vi "RT testbead.vi"() -> ()   [LabVIEW 2009]
uses:
  <vilib>/Instr/_visa.llb/VISA Configure Serial Port (Instr).vi
  behaviors/driveable path/drivable paths global.vi
panel:
  out "driveable path lengths (lines)":u16[](array[numeric])
  out "Serial Settings:Number of Bytes at Serial Port":u32
  in  "stop":bool
  out "read buffer":string
  in  "VISA resource name":refnum<visa-resource-name>
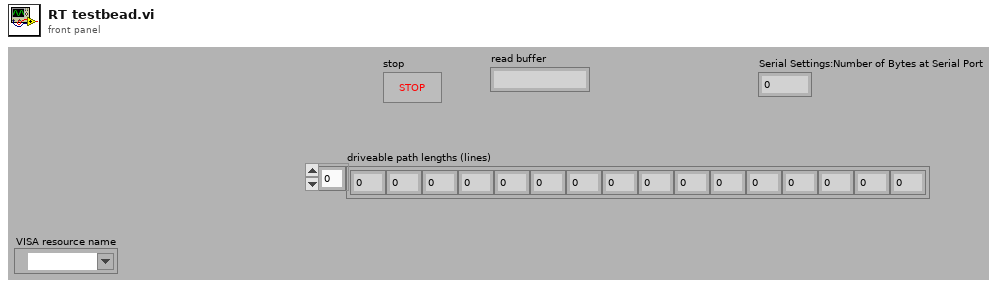
[diagram p1: front panel]
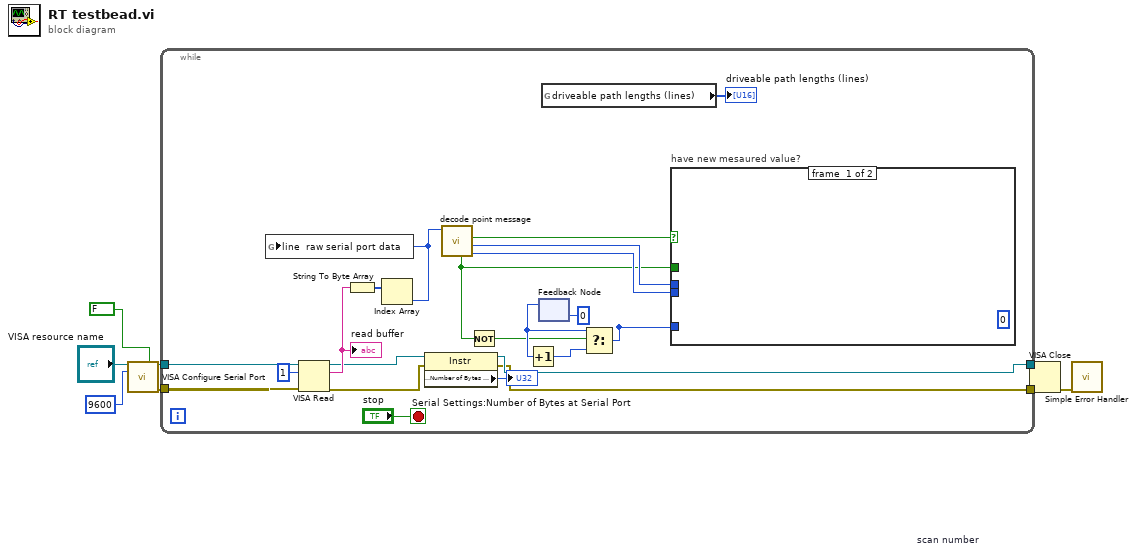
[diagram p0: block diagram]
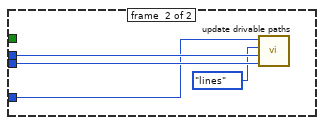
[diagram p2: hidden frame]
diagram:
  n1 = call-poly "VISA Configure Serial Port"("VISA resource name"="VISA resource name", "Enable Termination\nChar (T)"=FALSE ("Enable Termination\nChar (T)"), "baud rate (9600)"=u32 9600) -> ("VISA resource name out"=w4:refnum<visa-resource-name>, "error out"=w3:errorcluster)  [unwired: 11 in]
  n2 = while {
    tunnel: w4 -> [w30]
    tunnel: w3 -> [w29]
    tunnel: [w15] -> w2
    tunnel: [w13] -> w1
    stop <- "stop" stop-if-true
    n3 = VISA Read(VISA resource name=w30, byte count=u32 1, error in (no error)=w29) -> (VISA resource name out=w16:refnum<visa-resource-name>, read buffer=w26:string, error out=w14:errorcluster)  [unwired: 1 out]
    "read buffer" <- w26
    n4 = String To Byte Array(string=w26) -> (unsigned byte array=w25:u8[])
    n5 = Index Array(array=w25) -> (element=w17:u8)  [unwired: 1 in]
    n6 = global write "drivable paths global.vi" "line  raw serial port data"(w17) -> ()
    n7 = property class="Instr"(reference=w16, error in=w14) -> (reference out=w15:refnum<visa-resource-name>, error out=w13:errorcluster, "Serial Settings:Number of Bytes at Serial Port"=→"Serial Settings:Number of Bytes at Serial Port":u32)
    n8 = call "decode point message.vi"("input stream"=w17) -> ("y value"=w23:i16, "x value"=w24:i16, "new y"=w9:bool, "waiting for new message"=w11:bool)  [unwired: 6 in, 1 out]
    n9 = Not(x=w11) -> (.not. x?=w18:bool)
    n10 = feedback #1 "scan number"(u8 0 ("y")) -> (w20:u8)
    n11 = Increment(x=w20) -> (x+1=w21:u8)
    n12 = global read "drivable paths global.vi" "driveable path lengths (lines)"() -> (→"driveable path lengths (lines)":u16[])
    n13 = Select(t=w20, s=w18, f=w21) -> (s? t:f=w19:u8)
    n14 = case "have new mesaured value?" shown="True" w9 {
      tunnel: w11 -> [_ _]
      tunnel: w24 -> [_ w34]
      tunnel: w23 -> [_ w33]
      tunnel: w19 -> [_ w31]
      frame #0 {
        (unwired) u8 0 ("y")
      }
      frame #1 {
        n15 = call "update drivable paths.vi"("Robot Y"=w33, "Robot X"=w34, "update lines or objects"=enum16{"lines", "obstacles"}."lines", "Scan Number"=w31) -> ()  [unwired: 1 in]
      }
    }
  }
  n16 = VISA Close(VISA resource name=w2, error in (no error)=w1) -> (error out=w8:errorcluster)
  n17 = call <vilib>:"Simple Error Handler.vi"("error in (no error)"=w8) -> ()  [unwired: 4 in, 5 out]
